vi "Get Greeter_res.vi"(8 "error in (no error)":errorcluster, 11 "gRPCid":T1) -> (0 "error out":errorcluster, 2 "package_templatemessage":T2, 3 "gRPCid out":T1)   [LabVIEW 2019, in "Generated_server.lvlib"]
uses:
  Generated_server.lvlib
  Greeter_res.ctl
  Greeter_res_res_oneof/Greeter_res_res_oneof.lvclass
  <vilib>/gRPC/LabVIEW gRPC Library/Shared/grpcId.ctl
  Greeter_res_Flat.ctl
  Greeter_res_res_oneof/Greeter_res_res_oneof.lvclass/Greeter_res_res_oneof.ctl
  2ed25e12-861d-4677-8ead-ace2906b2041.vi
  <vilib>/gRPC/LabVIEW gRPC Library/Shared/TranslateGrpcError.vi
  Greeter_res_res_oneof/Setres_int32.vi
  Greeter_res_res_oneof/Setres_int64.vi
  Greeter_res_res_oneof/Setres_uint32.vi
  Greeter_res_res_oneof/Setres_uint64.vi
  Greeter_res_res_oneof/Setres_sint32.vi
  Greeter_res_res_oneof/Setres_sint64.vi
  Greeter_res_res_oneof/Setres_fixed32.vi
  Greeter_res_res_oneof/Setres_fixed64.vi
  Greeter_res_res_oneof/Setres_sfixed32.vi
  Greeter_res_res_oneof/Setres_sfixed64.vi
  Greeter_res_res_oneof/Setres_float.vi
  Greeter_res_res_oneof/Setres_double.vi
  Greeter_res_res_oneof/Setres_bool.vi
  Greeter_res_res_oneof/Setres_string.vi
  Greeter_res_res_oneof/Setres_bytes.vi
  <vilib>/gRPC/LabVIEW gRPC Library/Server API/Server/Get Server DLL Path.vi
  <vilib>/Utility/error.llb/Error Cluster From Error Code.vi
  <vilib>/Utility/error.llb/Simple Error Handler.vi
  Greeter_res_res_oneof/GetFieldFromProtobufIndexGreeter_res_res_oneof.vi
  <vilib>/gRPC/LabVIEW gRPC Library/grpc-lvsupport-release.lvlib
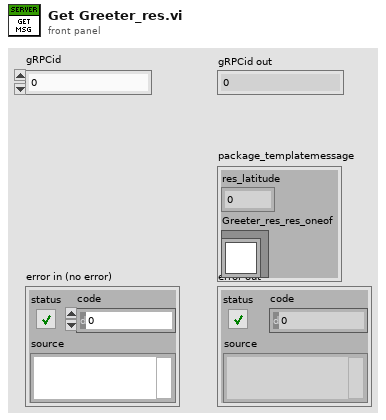
[diagram p1: front panel]
types:
  T1 = typedef "grpc-lvsupport-release.lvlib/grpcId.ctl" = u64
  T2 = typedef "Generated_server.lvlib/Greeter_res.ctl" = cluster{"res_latitude":i32, "Greeter_res_res_oneof":refnum<class "Greeter_res_res_oneof.lvclass">}
  T3 = typedef "Generated_server.lvlib/Greeter_res_Flat.ctl" = cluster{"res_latitude":i32, "Greeter_res_res_oneof_selected_index":i32, "res_int32":i32, "res_int64":i64, "res_uint32":u32, "res_uint64":u64, "res_sint32":i32, "res_sint64":i64, "res_fixed32":u32, "res_fixed64":u64, "res_sfixed32":i32, "res_sfixed64":i64, "res_float":sgl, "res_double":dbl, "res_bool":bool, "res_string":string, "res_bytes":u8[]}
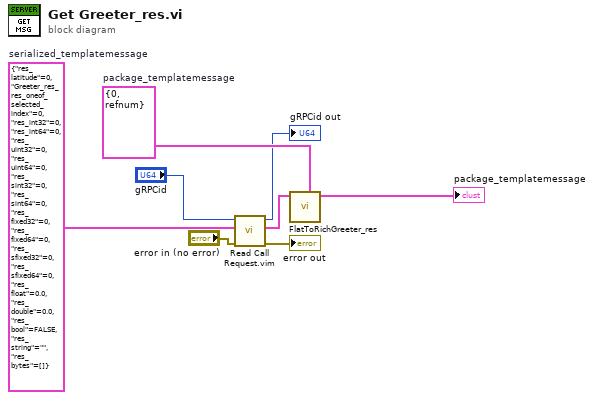
[diagram p0: block diagram]
diagram:
  w6 = T3 {"res_latitude"=0, "Greeter_res_res_oneof_selected_index"=0, "res_int32"=0, "res_int64"=0, "res_uint32"=0, "res_uint64"=0, "res_sint32"=0, "res_sint64"=0, "res_fixed32"=0, "res_fixed64"=0, "res_sfixed32"=0, "res_sfixed64"=0, "res_float"=0.0, "res_double"=0.0, "res_bool"=FALSE, "res_string"="", "res_bytes"=[]}  # serialized_templatemessage
  w5 = T2 {"res_latitude"=0, "Greeter_res_res_oneof"=refnum}  # package_templatemessage
  n1 = call "Read Call Request.vim"("error in"="error in (no error)", "Request Type"=w6, "gRPCid in"="gRPCid") -> ("error out"=→"error out":errorcluster, "Request Data"=w4:T3, "gRPCid out"=→"gRPCid out":T1)  [unwired: 6 in]
  n2 = call "FlatToRichGreeter_res.vi"("OutputClusterType"=w5, "InputCluster"=w4) -> ("OutputCluster"=→"package_templatemessage":T2)  [unwired: 9 in]
